vi "fmt_convertFormatString.vi"(8 "error in (no error)":errorcluster, 11 "format string":string) -> (0 "error out":errorcluster, 3 "format string out":string)   [LabVIEW 2020, in "NI_ExcelFile.lvlib"]
uses:
  <vilib>/express/express shared/NI_ExcelFile/NI_ExcelFile.lvlib
panel:
  out "errors":errorcluster[](array[cluster])
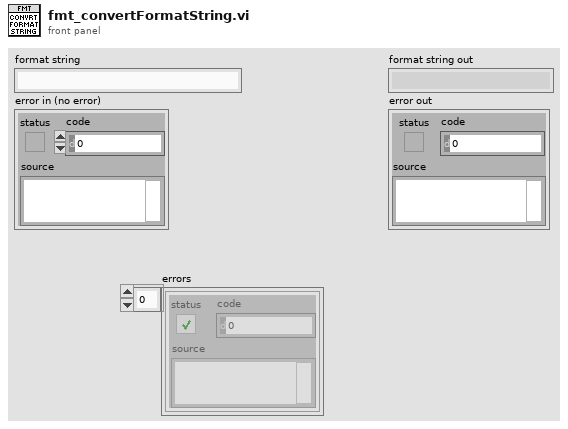
[diagram p1: front panel]
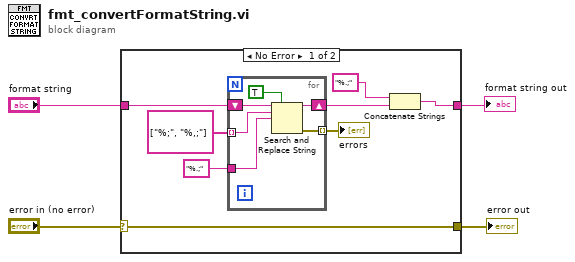
[diagram p0: block diagram]
diagram:
  n1 = case shown="No Error" "error in (no error)" {
    selector: "error in (no error)" -> [w10 w20]
    tunnel: "format string" -> [w9 w19]
    tunnel: [w11 w19] -> w3
    tunnel: [w10 w20] -> w1
    frame No Error {
      n2 = for {
        tunnel: string[] ["%;", "%,;"] -> [w17] mode=indexing
        shift-right: [w16] -> w7
        shift-left: w9 -> [w18]
        tunnel: "%.;" ("search string") -> [w14]
        tunnel: [w13] -> w5 mode=indexing
        n3 = Search and Replace String(replace all?=TRUE ("replace all? (F)"), input string=w18, search string=w17, replace string=w14) -> (result string=w16:string, error out=w13:errorcluster)  [unwired: 4 in, 2 out]
      }
      "errors" <- w5
      n4 = Concatenate Strings("%.;", w7) -> (w11:string)
    }
    frame Error {
    }
  }
  "format string out" <- w3
  "error out" <- w1
